vi "Write dvr.vi"(8 "error in (no error)":errorcluster, 10 "data value reference":refnum<data-value>, 11 "AbstractBattery in":refnum<class "AbstractBattery.lvclass">) -> (0 "error out":errorcluster, 3 "AbstractBattery out":refnum<class "AbstractBattery.lvclass">)   [LabVIEW 2011, in "AbstractBattery.lvclass"]
uses:
  AbstractBattery.lvclass
  AbstractBattery.lvclass/AbstractBattery.ctl
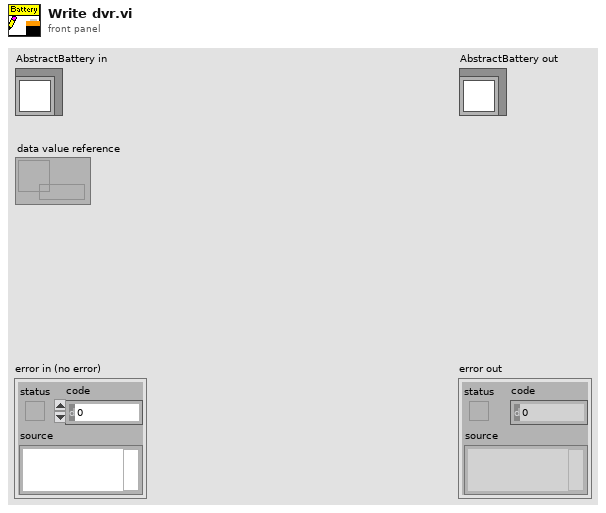
[diagram p1: front panel]
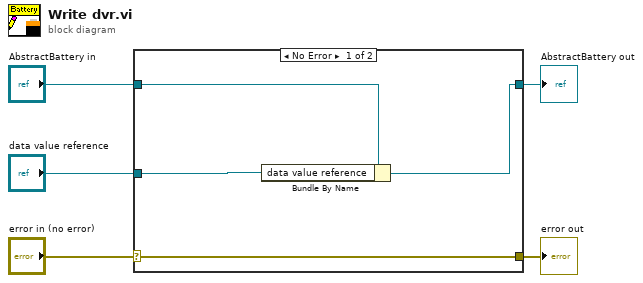
[diagram p0: block diagram]
diagram:
  n1 = case shown="No Error" "error in (no error)" {
    selector: "error in (no error)" -> [w9 w10]
    tunnel: [w9 w10] -> w4
    tunnel: [w7 w11] -> w2
    tunnel: "AbstractBattery in" -> [w8 w11]
    tunnel: "data value reference" -> [w6 _]
    frame No Error {
      n2 = Bundle By Name(cluster=w8, "data value reference"=w6) -> (w7:refnum<class "AbstractBattery.lvclass">)
    }
    frame Error {
    }
  }
  "error out" <- w4
  "AbstractBattery out" <- w2
